vi "SubVI_initdrivetalon.vi"(5 "PhaseSensor":bool, 7 "Invert?":bool, 8 "error in (no error)":errorcluster, 9 "Device Number":u8, 10 "TalonToFollow":T1={"DeviceStatus"={"status"=FALSE, "code"=0, "source"=""}, "Type"=enum."PWM", "PWM"={"PWM Channel"=enum."PWM 0", "DeadBand"={"Name"="", "maxPositivePwm"=0, "minPositivePwm"=0, "centerPwm"=0, "maxNegativePwm"=0, "minNegativePwm"=0, "angularRange"=0}}, "CAN"={"Device Number"=255, "SetOutput VI Ref"=variant, "GetOutput VI Ref"=variant, "Enable VI Ref"=variant, "Disable VI Ref"=variant, "Data"=variant}, "Invert"=FALSE, "DIO PWM"={"PWM \"Enable\" Channel"=enum."PWM 0", "DIOChannel"=enum."DIO 0", "PWM Rate"=0.0}}, 11 "refnum name":string="FrontLeftTalon") -> (0 "error out":errorcluster, 3 "PhoenixMotorControlDevRef":T1)   [LabVIEW 2017]
uses:
  <vilib>/Rock Robotics/WPI/MotorControl/WPI_MotorControlDeviceRef.ctl
  <vilib>/Rock Robotics/WPI/MotorControl/WPI_MotorControlType.ctl
  <vilib>/Rock Robotics/SystemInterfaces/DIO/FPGA_DIOPWMChannel.ctl
  <vilib>/Rock Robotics/WPI/PWM/WPI_PWMDeadband.ctl
  <vilib>/Rock Robotics/SystemInterfaces/DIO/FPGA_DIOChannel.ctl
  <vilib>/Rock Robotics/WPI/ThirdParty/Phoenix-LabVIEW/Motor Controller/Controls/CTRE_Phoenix_MotorControl_FeedbackDevice.ctl
  <vilib>/Rock Robotics/WPI/ThirdParty/Phoenix-LabVIEW/Motor Controller/Controls/CTRE_Phoenix_MotorControl_SensorTermFeedbackDevice_Enhanced.ctl
  Constants.vi
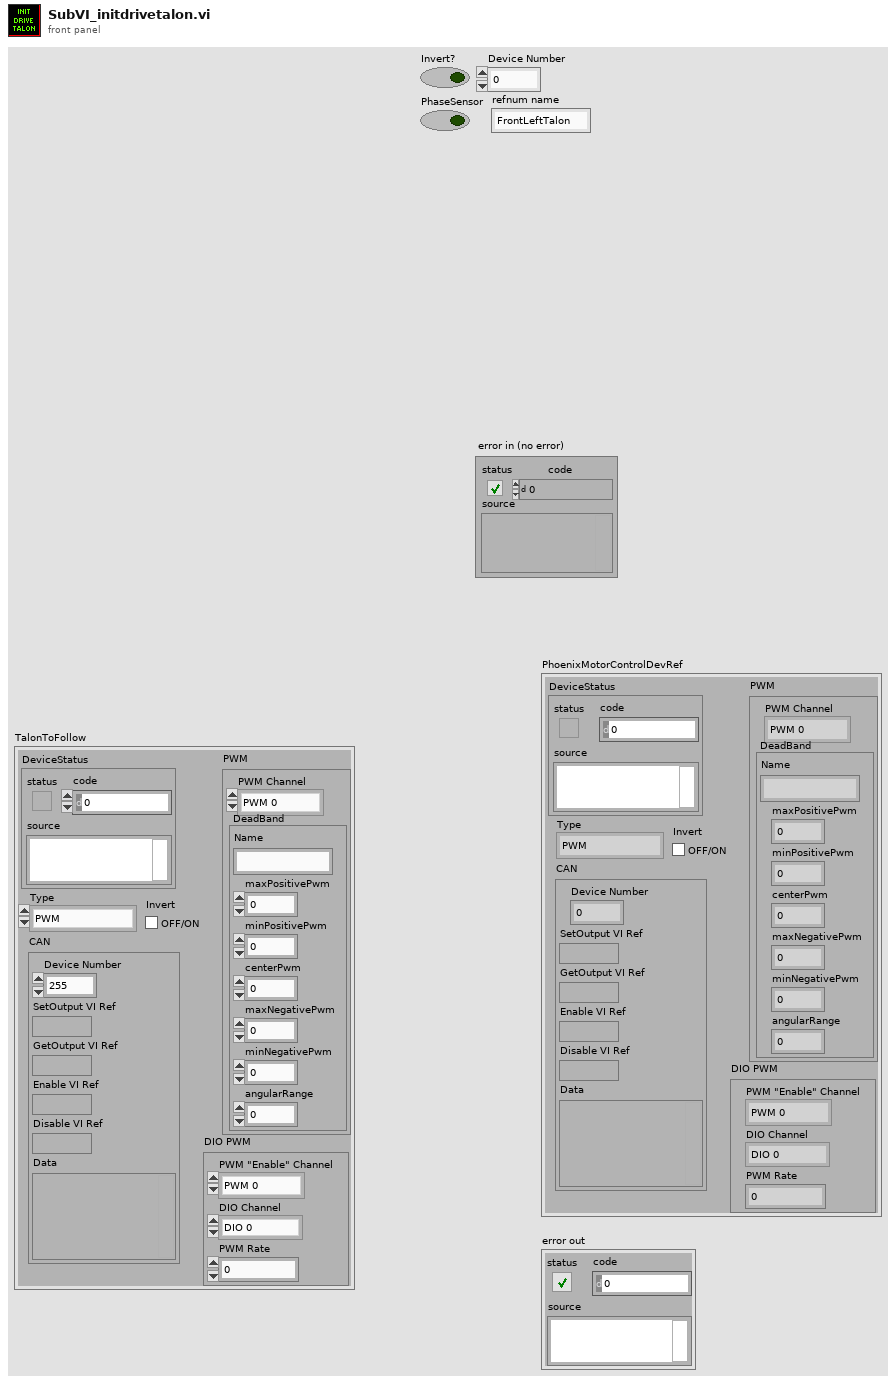
[diagram p1: front panel]
types:
  T1 = typedef "WPI_MotorControlDeviceRef.ctl" = cluster{"DeviceStatus":errorcluster, "Type":T2, "PWM":cluster{"PWM Channel":T3, "DeadBand":T4}, "CAN":cluster{"Device Number":u8, "SetOutput VI Ref":variant, "GetOutput VI Ref":variant, "Enable VI Ref":variant, "Disable VI Ref":variant, "Data":variant}, "Invert":bool, "DIO PWM":cluster{"PWM \"Enable\" Channel":T3, "DIOChannel":T5, "PWM Rate":dbl}}
  T2 = typedef "WPI_MotorControlType.ctl" = enum16{"PWM", "CAN", "DIO PWM"}
  T3 = typedef "FPGA_DIOPWMChannel.ctl" = enum8{"PWM 0", "PWM 1", "PWM 2", "PWM 3", "PWM 4", "PWM 5", "PWM 6", "PWM 7", "PWM 8", "PWM 9", "PWM MXP 0", "PWM MXP 1", "PWM MXP 2", "PWM MXP 3", "PWM MXP 4", "PWM MXP 5", "PWM MXP 6", "PWM MXP 7", "PWM MXP 8", "PWM MXP 9", "Invalid"}
  T4 = typedef "WPI_PWMDeadband.ctl" = cluster{"Name":string, "maxPositivePwm":i32, "minPositivePwm":i32, "centerPwm":i32, "maxNegativePwm":i32, "minNegativePwm":i32, "angularRange":u16}
  T5 = typedef "FPGA_DIOChannel.ctl" = enum8{"DIO 0", "DIO 1", "DIO 2", "DIO 3", "DIO 4", "DIO 5", "DIO 6", "DIO 7", "DIO 8", "DIO 9", "DIO MXP 0", "DIO MXP 1", "DIO MXP 2", "DIO MXP 3", "DIO MXP 4", "DIO MXP 5", "DIO MXP 6", "DIO MXP 7", "DIO MXP 8", "DIO MXP 9", "DIO MXP 10", "DIO MXP 11", "DIO MXP 12", "DIO MXP 13", "DIO MXP 14", "DIO MXP 15", "SPI Port CS1", "SPI Port CS2", "SPI Port CS3", "SPI Port MISO", "SPI Port MOSI", "Invalid"}
  T6 = typedef "CTRE_Phoenix_MotorControl_FeedbackDevice.ctl" = i8
  T7 = typedef "TypeDef_PIDFgains.ctl" = cluster{"kP":dbl, "kI ":dbl, "kD":dbl, "kF":dbl, "I Zone":dbl, "Peak Out":dbl}
  T8 = typedef "CTRE_Phoenix_MotorControl_SensorTermFeedbackDevice_Enhanced.ctl" = i8
  T9 = typedef "CTRE_Phoenix_MotorControl_RemoteSourceType.ctl" = enum16{"Off", "Talon SRX Selected Sensor", "Pigeon IMU Yaw", "Pigeon IMU Pitch", "Pigeon IMU Roll", "CANifier Quadrature", "CANifier PWM Input 0", "CANifier PWM Input 1", "CANifier PWM Input 2", "CANifier PWM Input 3", "Gadgeteer Pigeon Yaw", "Gadgeteer Pigeon Pitch", "Gadgeteer Pigeon Roll"}
  T10 = cluster{"left talon":i32, "left victor 0":i32, "left victor 1":i32, "right talon":i32, "right victor 0":i32, "right victor 1":i32, "pigeon":i32}
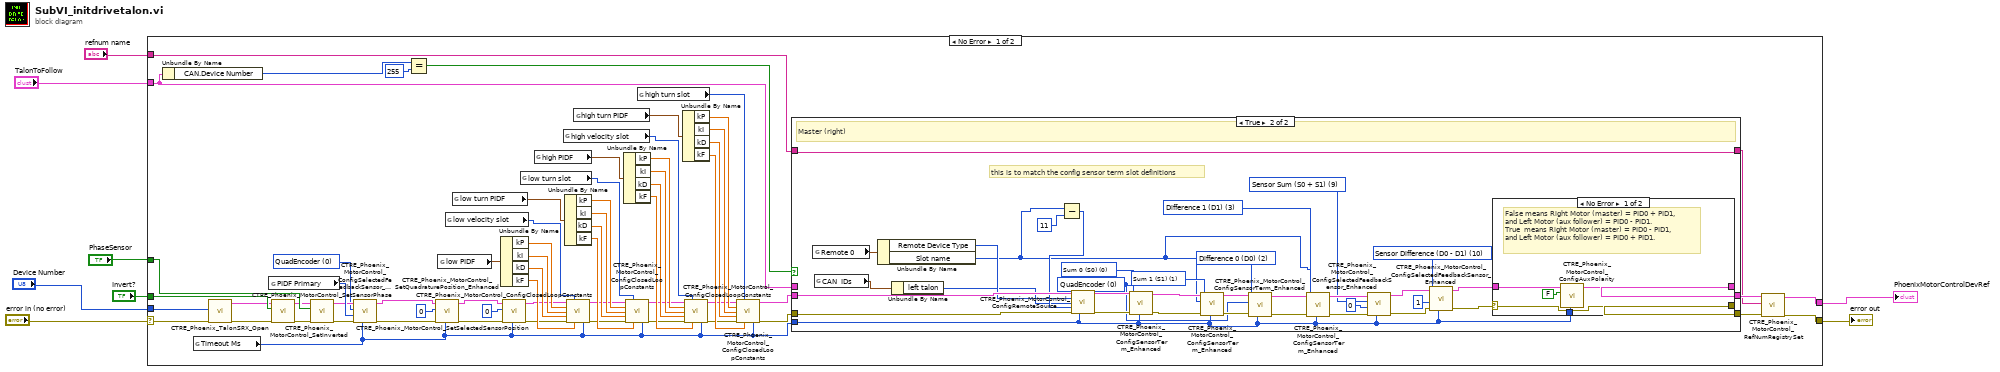
[diagram p0: block diagram]
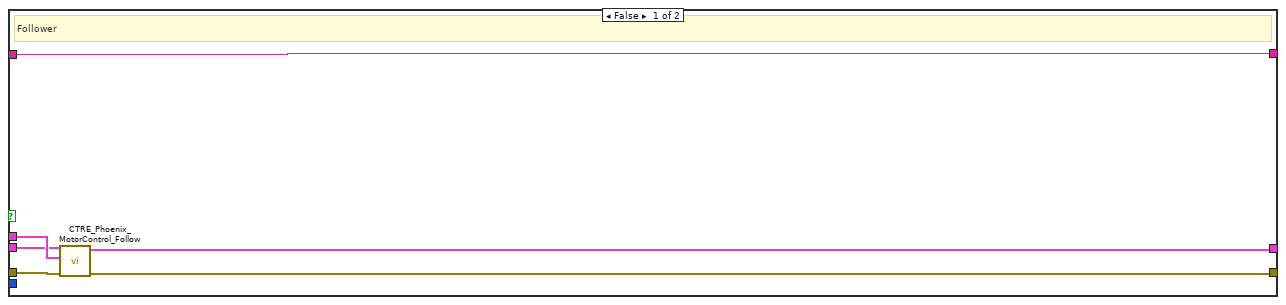
[diagram p2: hidden frame]
diagram:
  n1 = case shown="No Error" "error in (no error)" {
    selector: "error in (no error)" -> [w67 w121]
    tunnel: "refnum name" -> [w71 _]
    tunnel: "Invert?" -> [w70 _]
    tunnel: "PhaseSensor" -> [w69 _]
    tunnel: "Device Number" -> [w68 _]
    tunnel: [w12 w121] -> w3
    tunnel: [w11 _] -> w2
    tunnel: "TalonToFollow" -> [w63 _]
    frame No Error {
      w19 = T6 0 items=["None"=-1, "QuadEncoder"=0, "Analog"=2, "Tachometer"=4, "Pulse Width Encoded Position"=8, "Sensor Sum (S0 + S1)"=9, "Sensor Difference (D0 - D1)"=10, "Remote Source 0"=11, "Remote Source 1"=12, "Software Emulated"=15] ("Feedback Device")
      n2 = Unbundle By Name(w63) -> ("CAN.Device Number"=w66:u8)
      n3 = global read "Constants.vi" "Timeout Ms"() -> (w9:i32)
      n4 = call <vilib>:"CTRE_Phoenix_TalonSRX_Open.vi"("error in"=w67, "Device Number"=w68) -> ("error out"=w27:errorcluster, "CAN Talon SRX Ref"=w24:T1)  [unwired: 8 in]
      n5 = global read "Constants.vi" "PIDF Primary"() -> (w58:i32)
      n6 = call <vilib>:"CTRE_Phoenix_MotorControl_SetInverted.vi"("error in (no error)"=w27, "Invert?"=w70, "PhoenixMotorControlDevRef"=w24) -> ("error out"=w28:errorcluster, "PhoenixMotorControlDevRef"=w25:T1)  [unwired: 7 in]
      n7 = call <vilib>:"CTRE_Phoenix_MotorControl_SetSensorPhase.vi"("error in (no error)"=w28, "PhaseSensor"=w69, "PhoenixMotorControlDevRef"=w25) -> ("error out"=w29:errorcluster, "PhoenixMotorControlDevRef"=w26:T1)  [unwired: 7 in]
      n8 = call <vilib>:"CTRE_Phoenix_MotorControl_ConfigSelectedFeedbackSensor_Enhanced.vi"("timeoutMs"=w9, "error in (no error)"=w29, "pidLoopIdx"=w58, "Feedback Device"=w19, "PhoenixMotorControlDevRef"=w26) -> ("error out"=w23:errorcluster, "PhoenixMotorControlDevRef"=w22:T1)  [unwired: 5 in]
      n9 = Equal?(x=w66, y=u8 255) -> (x = y?=w64:bool)
      n10 = call <vilib>:"CTRE_Phoenix_MotorControl_SetQuadraturePosition_Enhanced.vi"("timeoutMs"=w9, "error in (no error)"=w23, "New Position"=0, "PhoenixMotorControlDevRef"=w22) -> ("error out"=w21:errorcluster, "PhoenixMotorControlDevRef"=w20:T1)  [unwired: 6 in]
      n11 = global read "Constants.vi" "low PIDF"() -> (w42:T7)
      n12 = global read "Constants.vi" "low velocity slot"() -> (w38:i32)
      n13 = global read "Constants.vi" "low turn PIDF"() -> (w46:T7)
      n14 = Unbundle By Name(w42) -> ("kP"=w43:dbl, "kI"=w44:dbl, "kD"=w45:dbl, "kF"=w59:dbl)
      n15 = call <vilib>:"CTRE_Phoenix_MotorControl_SetSelectedSensorPosition.vi"("timeoutMs"=w9, "error in (no error)"=w21, "New Sensor Position"=0, "PhoenixMotorControlDevRef"=w20) -> ("error out"=w33:errorcluster, "PhoenixMotorControlDevRef"=w32:T1)  [unwired: 6 in]
      n16 = global read "Constants.vi" "low turn slot"() -> (w39:i32)
      n17 = global read "Constants.vi" "high PIDF"() -> (w50:T7)
      n18 = global read "Constants.vi" "high velocity slot"() -> (w40:i32)
      n19 = Unbundle By Name(w46) -> ("kP"=w47:dbl, "kI"=w48:dbl, "kD"=w49:dbl, "kF"=w60:dbl)
      n20 = call <vilib>:"CTRE_Phoenix_MotorControl_ConfigClosedLoopConstants.vi"("PhoenixMotorControlDevRef"=w32, "slotIdx"=w38, "P"=w43, "I"=w44, "D"=w45, "error in (no error)"=w33, "F"=w59, "timeoutMs"=w9) -> ("PhoenixMotorControlDevRef"=w37:T1, "error out"=w34:errorcluster)  [unwired: 6 in]
      n21 = global read "Constants.vi" "high turn PIDF"() -> (w54:T7)
      n22 = Unbundle By Name(w50) -> ("kP"=w51:dbl, "kI"=w52:dbl, "kD"=w53:dbl, "kF"=w61:dbl)
      n23 = call <vilib>:"CTRE_Phoenix_MotorControl_ConfigClosedLoopConstants.vi"("PhoenixMotorControlDevRef"=w37, "slotIdx"=w39, "P"=w47, "I"=w48, "D"=w49, "error in (no error)"=w34, "F"=w60, "timeoutMs"=w9) -> ("PhoenixMotorControlDevRef"=w36:T1, "error out"=w35:errorcluster)  [unwired: 6 in]
      n24 = global read "Constants.vi" "high turn slot"() -> (w41:i32)
      n25 = Unbundle By Name(w54) -> ("kP"=w55:dbl, "kI"=w56:dbl, "kD"=w57:dbl, "kF"=w62:dbl)
      n26 = call <vilib>:"CTRE_Phoenix_MotorControl_ConfigClosedLoopConstants.vi"("PhoenixMotorControlDevRef"=w36, "slotIdx"=w40, "P"=w51, "I"=w52, "D"=w53, "error in (no error)"=w35, "F"=w61, "timeoutMs"=w9) -> ("PhoenixMotorControlDevRef"=w31:T1, "error out"=w30:errorcluster)  [unwired: 6 in]
      n27 = call <vilib>:"CTRE_Phoenix_MotorControl_ConfigClosedLoopConstants.vi"("PhoenixMotorControlDevRef"=w31, "slotIdx"=w41, "P"=w55, "I"=w56, "D"=w57, "error in (no error)"=w30, "F"=w62, "timeoutMs"=w9) -> ("PhoenixMotorControlDevRef"=w16:T1, "error out"=w15:errorcluster)  [unwired: 6 in]
      n28 = case shown="True" w64 {
        tunnel: w71 -> [w72 w111]
        tunnel: w63 -> [w77 _]
        tunnel: w16 -> [w76 w113]
        tunnel: w15 -> [w75 w112]
        tunnel: [w73 w79] -> w14
        tunnel: [w74 w81] -> w13
        tunnel: [w72 w111] -> w10
        tunnel: w9 -> [_ w78]
        frame False {
          # "Follower"
          n29 = call <vilib>:"CTRE_Phoenix_MotorControl_Follow.vi"("error in (no error)"=w75, "Master Controller to Follow"=w77, "PhoenixMotorControlDevRef"=w76) -> ("error out"=w73:errorcluster, "PhoenixMotorControlDevRef"=w74:T1)  [unwired: 7 in]
        }
        frame True {
          w85 = T6 10 items=["None"=-1, "QuadEncoder"=0, "Analog"=2, "Tachometer"=4, "Pulse Width Encoded Position"=8, "Sensor Sum (S0 + S1)"=9, "Sensor Difference (D0 - D1)"=10, "Remote Source 0"=11, "Remote Source 1"=12, "Software Emulated"=15] ("Feedback Device")
          w88 = T6 9 items=["None"=-1, "QuadEncoder"=0, "Analog"=2, "Tachometer"=4, "Pulse Width Encoded Position"=8, "Sensor Sum (S0 + S1)"=9, "Sensor Difference (D0 - D1)"=10, "Remote Source 0"=11, "Remote Source 1"=12, "Software Emulated"=15] ("Feedback Device")
          w91 = u16 3 items=["Sum 0 (S0)", "Sum 1 (S1)", "Difference 0 (D0)", "Difference 1 (D1)"] ("Sensor Term")
          w93 = u16 2 items=["Sum 0 (S0)", "Sum 1 (S1)", "Difference 0 (D0)", "Difference 1 (D1)"] ("Sensor Term")
          w102 = u16 1 items=["Sum 0 (S0)", "Sum 1 (S1)", "Difference 0 (D0)", "Difference 1 (D1)"] ("Sensor Term")
          w94 = T8 0 items=["None"=-1, "QuadEncoder"=0, "Analog"=2, "Tachometer"=4, "Pulse Width Encoded Position"=8, "Remote Source 0"=11, "Remote Source 1"=12, "Software Emulated"=15] ("Feedback Device")
          w105 = u16 0 items=["Sum 0 (S0)", "Sum 1 (S1)", "Difference 0 (D0)", "Difference 1 (D1)"] ("Sensor Term")
          # "this is to match the config sensor term slot definitions"
          # "Master (right)"
          n30 = global read "Constants.vi" "Remote 0"() -> (w109:cluster{"Remote Device Type":T9, "Slot name":T8})
          n31 = global read "Constants.vi" "CAN  IDs"() -> (w110:T10)
          n32 = Unbundle By Name(w109) -> ("Remote Device Type"=w108:T9, "Slot name"=w92:T8)
          n33 = Unbundle By Name(w110) -> ("left talon"=w99:i32)
          n34 = Subtract(x=w92, y=11) -> (x-y=w100:i32)
          n35 = call <vilib>:"CTRE_Phoenix_MotorControl_ConfigRemoteSource.vi"("PhoenixMotorControlDevRef"=w113, "Remote Device Type"=w108, "Remote Device ID"=w99, "Source Index (0/1)"=w100, "error in (no error)"=w112, "timeoutMs"=w78) -> ("PhoenixMotorControlDevRef"=w107:T1, "error out"=w106:errorcluster)  [unwired: 8 in]
          n36 = call <vilib>:"CTRE_Phoenix_MotorControl_ConfigSensorTerm_Enhanced.vi"("timeoutMs"=w78, "error in (no error)"=w106, "Sensor Term"=w105, "Feedback Device"=w94, "PhoenixMotorControlDevRef"=w107) -> ("error out"=w103:errorcluster, "PhoenixMotorControlDevRef"=w104:T1)  [unwired: 5 in]
          n37 = call <vilib>:"CTRE_Phoenix_MotorControl_ConfigSensorTerm_Enhanced.vi"("timeoutMs"=w78, "error in (no error)"=w103, "Sensor Term"=w102, "Feedback Device"=w92, "PhoenixMotorControlDevRef"=w104) -> ("error out"=w97:errorcluster, "PhoenixMotorControlDevRef"=w98:T1)  [unwired: 5 in]
          n38 = call <vilib>:"CTRE_Phoenix_MotorControl_ConfigSensorTerm_Enhanced.vi"("timeoutMs"=w78, "error in (no error)"=w97, "Sensor Term"=w93, "Feedback Device"=w94, "PhoenixMotorControlDevRef"=w98) -> ("error out"=w95:errorcluster, "PhoenixMotorControlDevRef"=w96:T1)  [unwired: 5 in]
          n39 = call <vilib>:"CTRE_Phoenix_MotorControl_ConfigSensorTerm_Enhanced.vi"("timeoutMs"=w78, "error in (no error)"=w95, "Sensor Term"=w91, "Feedback Device"=w92, "PhoenixMotorControlDevRef"=w96) -> ("error out"=w89:errorcluster, "PhoenixMotorControlDevRef"=w90:T1)  [unwired: 5 in]
          n40 = call <vilib>:"CTRE_Phoenix_MotorControl_ConfigSelectedFeedbackSensor_Enhanced.vi"("timeoutMs"=w78, "error in (no error)"=w89, "pidLoopIdx"=0, "Feedback Device"=w88, "PhoenixMotorControlDevRef"=w90) -> ("error out"=w83:errorcluster, "PhoenixMotorControlDevRef"=w84:T1)  [unwired: 5 in]
          n41 = call <vilib>:"CTRE_Phoenix_MotorControl_ConfigSelectedFeedbackSensor_Enhanced.vi"("timeoutMs"=w78, "error in (no error)"=w83, "pidLoopIdx"=1, "Feedback Device"=w85, "PhoenixMotorControlDevRef"=w84) -> ("error out"=w80:errorcluster, "PhoenixMotorControlDevRef"=w82:T1)  [unwired: 5 in]
          n42 = case shown="No Error" w80 {
            selector: w80 -> [w116 w120]
            tunnel: w82 -> [w118 w119]
            tunnel: [w117 w119] -> w81
            tunnel: [w116 w120] -> w79
            tunnel: w78 -> [w114 _]
            frame No Error {
              # "False means Right Motor (master) = PID0 + PID1, \nand Left Motor (aux follower) = PID0 - PID1.\nTrue  means Right Motor (master) = PID0 - PID1, \nand Left Motor (aux follower) = PID0 + PID1."
              n43 = call <vilib>:"CTRE_Phoenix_MotorControl_ConfigAuxPolarity.vi"("timeoutMs"=w114, "Invert"=FALSE, "PhoenixMotorControlDevRef"=w118) -> ("PhoenixMotorControlDevRef"=w117:T1)  [unwired: 8 in]
            }
            frame Error {
            }
          }
        }
      }
      n44 = call <vilib>:"CTRE_Phoenix_MotorControl_RefNumRegistrySet.vi"("error in (no error)"=w14, "refnum name"=w10, "PhoenixMotorControlDevRef"=w13) -> ("error out"=w12:errorcluster, "PhoenixMotorControlDevRef"=w11:T1)  [unwired: 7 in]
    }
    frame Error {
    }
  }
  "PhoenixMotorControlDevRef" <- w2
  "error out" <- w3
